vi "GOOP400_RemoveUnwantedChars.vi"(10 "StringIn":string) -> (2 "StringOut":string)   [LabVIEW 2014]
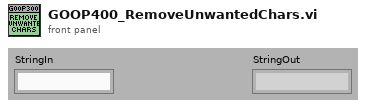
[diagram p1: front panel]
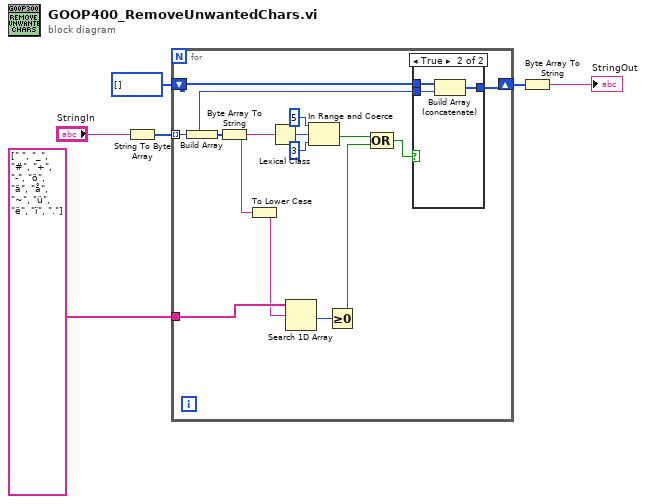
[diagram p0: block diagram]
diagram:
  n1 = String To Byte Array(string="StringIn") -> (unsigned byte array=w6:u8[])
  n2 = for {
    tunnel: w6 -> [w13] mode=indexing
    shift-right: [w14] -> w4
    shift-left: u8[] [] -> [w15]
    tunnel: string[] [" ", "_", "#", "+", "-", "ö", "ä", "å", "~", "ü", "ë", "ï", "."] ("1D array") -> [w11]
    n3 = Build Array(w13) -> (w18:u8[])
    n4 = Byte Array To String(unsigned byte array=w18) -> (string=w9:string)
    n5 = To Lower Case(string=w9) -> (all lower case string=w8:string)
    n6 = Lexical Class(1:w9) -> (0:w16:i16)
    n7 = Search 1D Array(1D array=w11, element=w8) -> (index of element=w10:i32)  [unwired: 1 in]
    n8 = In Range and Coerce(upper limit=i16 5, x=w16, lower limit=i16 3) -> (In Range?=w17:bool)  [unwired: 1 out]
    n9 = Greater Or Equal To 0?(x=w10) -> (x >= 0?=w7:bool)
    n10 = Compound Arithmetic op=OR(w17, w7) -> (w12:bool)
    n11 = case shown="True" w12 {
      tunnel: w15 -> [w21 w24]
      tunnel: [w21 w23] -> w14
      tunnel: w13 -> [_ w22]
      frame False {
      }
      frame True {
        n12 = Build Array (concatenate)(w24, w22) -> (w23:u8[])
      }
    }
  }
  n13 = Byte Array To String(unsigned byte array=w4) -> (string=→"StringOut":string)
